vi "KoherasStatus.vi"() -> ()   [LabVIEW 2013]
panel:
  in  "KoherasStatus":string
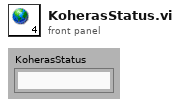
[diagram p1: front panel]
diagram:
